vi "Historico.vi"(0 "selected path in":path, 1 "CH?":T1(ring) caption="Seleccionar canal", 2 "Hystory":bool caption="Historico", 5 "Error In":errorcluster) -> (14 "Waveform Chart":dbl[](graph), 16 "string":string caption="Ultima Vista", 19 "Error Out":errorcluster)   [LabVIEW 2013]
uses:
  <vilib>/Utility/file.llb/Read From Spreadsheet File (DBL).vi
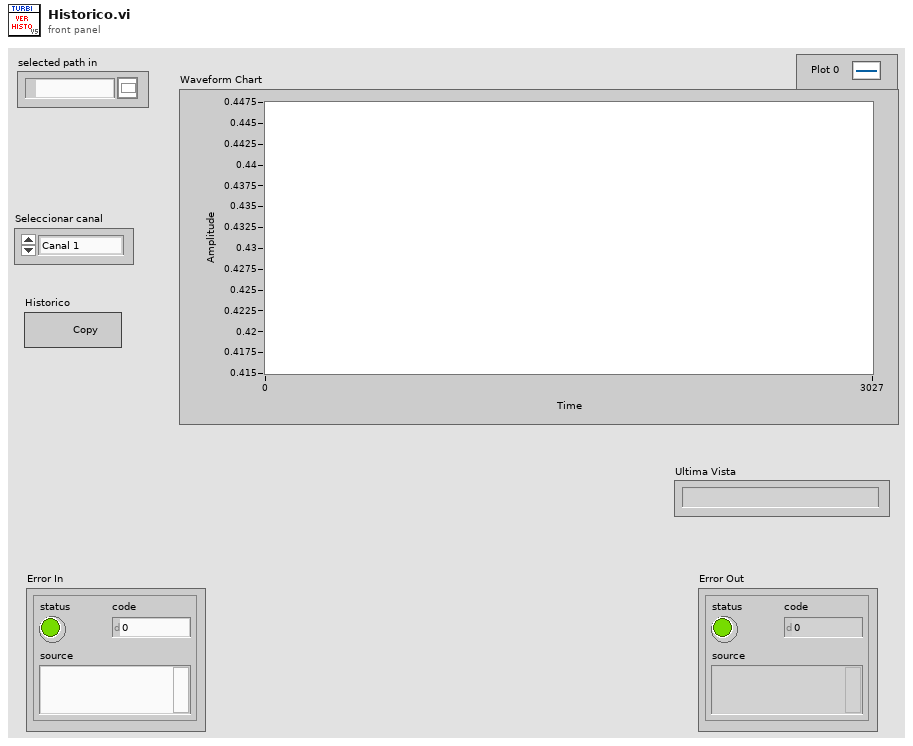
[diagram p1: front panel]
types:
  T1 = enum16{"Canal 1", "Canal 2", "Canal 3", "Canal 4", "Canal 5", "Canal 6", "Canal 7", "Canal 8"}
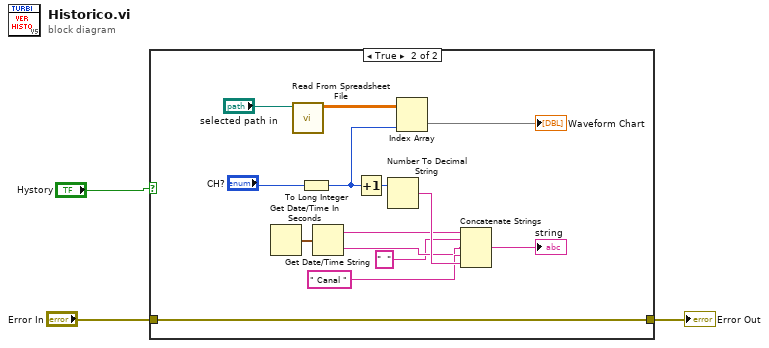
[diagram p0: block diagram]
diagram:
  n1 = case shown="True" "Hystory" {
    tunnel: [w4 w6] -> w3
    tunnel: "Error In" -> [w4 w6]
    frame False {
    }
    frame True {
      n2 = Get Date/Time In Seconds() -> (seconds since 1Jan1904=w8:timestamp)
      n3 = call-poly <vilib>:"Read From Spreadsheet File.vi"("file path (dialog if empty)"="selected path in") -> ("all rows"=w16:dbl[][])  [unwired: 6 in, 4 out]
      n4 = To Long Integer(number="CH?") -> (32bit integer=w5:i32)
      n5 = Get Date/Time String(seconds (now)=w8) -> (date string=w9:string, time string=w13:string)  [unwired: 2 in]
      n6 = Increment(x=w5) -> (x+1=w10:i32)
      n7 = Number To Decimal String(number=w10) -> (decimal integer string=w15:string)  [unwired: 1 in]
      n8 = Index Array(array=w16, index (col)=w5) -> (element=→"Waveform Chart":dbl[])  [unwired: 1 in]
      n9 = Concatenate Strings(w9, "  " ("string"), w13, " Canal " ("string"), w15) -> (→"string":string)
    }
  }
  "Error Out" <- w3
